vi "FEA_Model_Eigensolution.vi"(8 "error in (no error)":errorcluster, 11 "FEA_Model in":refnum<class "FEA_Model.lvclass">) -> (0 "error out":errorcluster, 3 "FEA_Model out":refnum<class "FEA_Model.lvclass">)   [LabVIEW 2021, in "FEA_Model.lvclass"]
uses:
  FEA_Model.lvclass
  FEA_Model.lvclass/FEA_Model.ctl
  <vilib>/Analysis/7linalg.llb/Eigenvalue and Vectors Output Option.ctl
  <vilib>/Analysis/baseanly.llb/Matrix Type of Inverse Matrix.ctl
  <vilib>/Analysis/7linalg.llb/Real Cholesky Factorization.vi
  <vilib>/Analysis/7linalg.llb/Real Generalized Eigenvalues and Vectors.vi
  <vilib>/Analysis/baseanly.llb/Full Cholesky Factorization.vi
  <vilib>/Analysis/baseanly.llb/Full Real Matrix Cholesky Factorization.vi
  <vilib>/Analysis/Matrix/Numeric/Conversions/Array To Matrix - RA2.vi
  <vilib>/Analysis/baseanly.llb/Real Inverse Matrix.vi
  <vilib>/Analysis/Matrix/Numeric/Multiply/Multiply - RM,RM.vi
  <vilib>/Analysis/Matrix/Numeric/Add/Add - RM,RM.vi
  <vilib>/Analysis/7linalg.llb/Real Eigenvalues and Vectors.vi
  <vilib>/Analysis/NI_AALPro.lvlib
  <vilib>/Analysis/Matrix/NI_Matrix.lvlib
  <vilib>/Analysis/NI_AALBase.lvlib
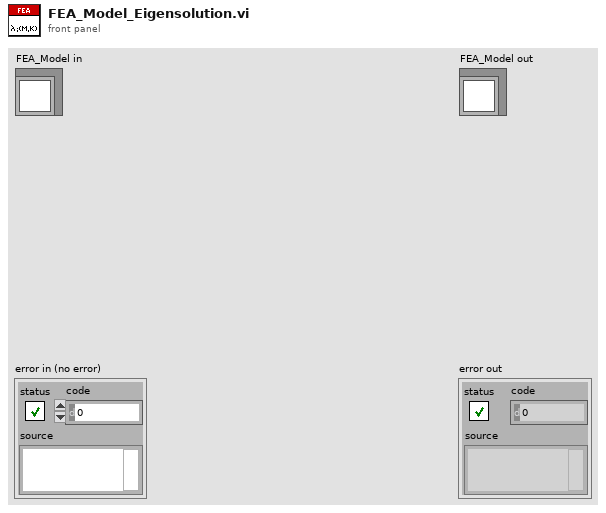
[diagram p1: front panel]
types:
  T1 = typedef "NI_AALBase.lvlib/Matrix Type of Inverse Matrix.ctl" = enum32{"General", "Positive Definite", "Lower Triangular", "Upper Triangular"}
  T2 = enum16{"LabVIEW Cholesky", "LabVIEW General", "LabVIEW Inverse", "LEMP"}
  T3 = typedef "NI_AALPro.lvlib/Eigenvalue and Vectors Output Option.ctl" = i32
  T4 = typedef "NI_Matrix.lvlib/RealMatrix.ctl" = dbl[][]
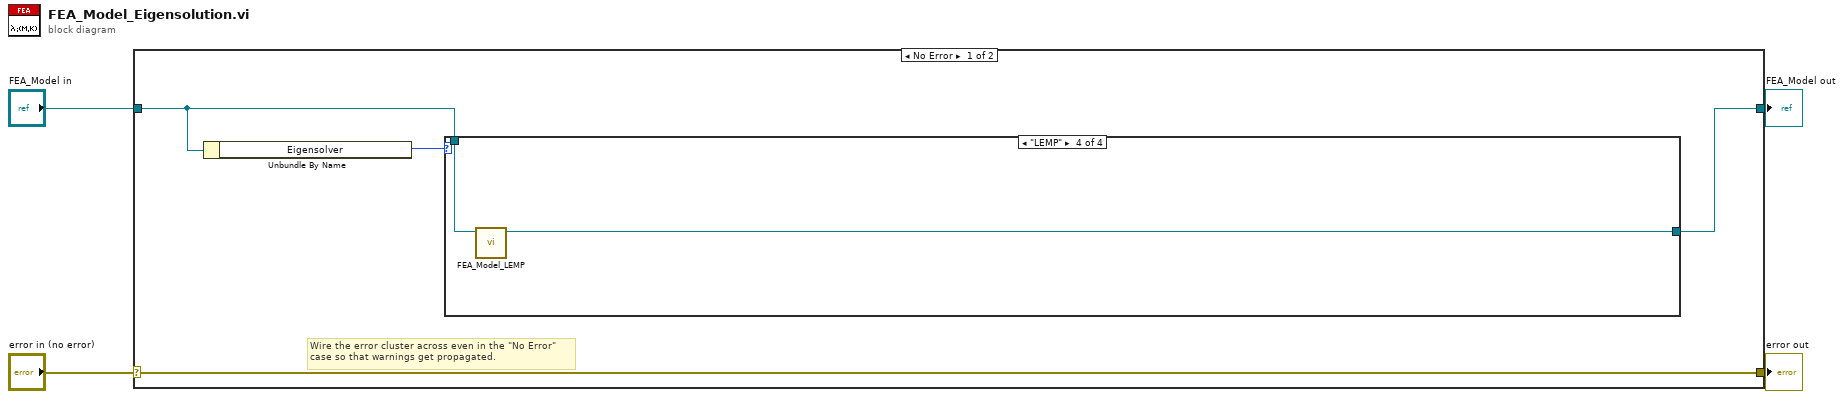
[diagram p0: block diagram]
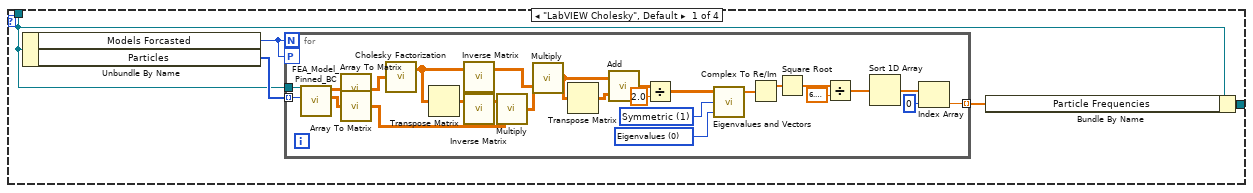
[diagram p2: hidden frame]
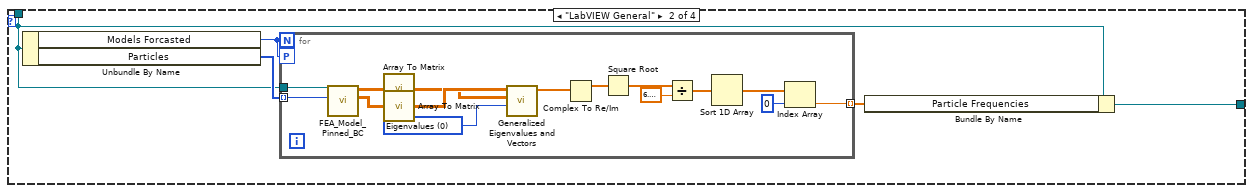
[diagram p3: hidden frame]
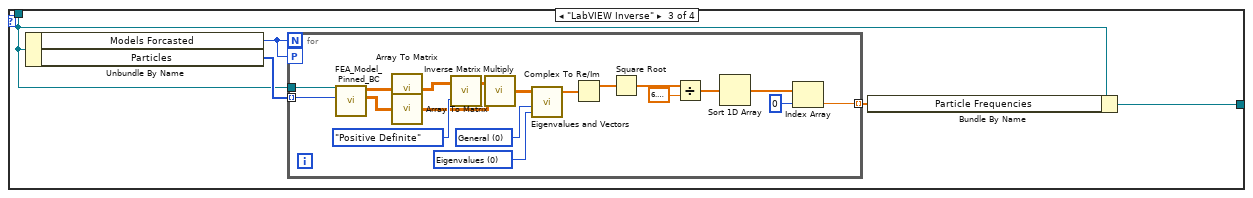
[diagram p4: hidden frame]
diagram:
  n1 = case shown="No Error" "error in (no error)" {
    selector: "error in (no error)" -> [w8 w87]
    tunnel: [w8 w87] -> w3
    tunnel: [w6 w86] -> w1
    tunnel: "FEA_Model in" -> [w5 w86]
    frame No Error {
      # "Wire the error cluster across even in the \"No Error\"\ncase so that warnings get propagated."
      n2 = Unbundle By Name(w5) -> ("Eigensolver"=w7:T2)
      n3 = case shown="\"LEMP\"" w7 {
        tunnel: [w10 w42 w61 w85] -> w6
        tunnel: w5 -> [w9 w40 w60 w84]
        frame "LabVIEW Cholesky", Default {
          n4 = Unbundle By Name(w9) -> ("Models Forcasted"=w13:i32, "Particles"=w12:i32[])
          n5 = for {
            N: w13 -> [_]
            workers-P: w13 -> [_]
            tunnel: w9 -> [w39]
            tunnel: w12 -> [w38] mode=indexing
            tunnel: [w29] -> w11 mode=indexing
            w18 = T3 0 items=["Eigenvalues", "Eigenvalues & Vectors"] ("output option")
            w19 = 1 items=["General", "Symmetric"] ("matrix type")
            n6 = call "FEA_Model_Pinned_BC.vi"("Pin Location"=w38, "FEA_Model in"=w39) -> ("K Matrix"=w36:dbl[][], "M Matrix"=w37:dbl[][])  [unwired: 8 in]
            n7 = call-poly <vilib>:"Array To Matrix.vi"("Real 2D Array"=w37) -> ("Real Matrix"=w16:T4)
            n8 = call-poly <vilib>:"Array To Matrix.vi"("Real 2D Array"=w36) -> ("Real Matrix"=w15:T4)
            n9 = call-poly <vilib>:"Cholesky Factorization.vi"("A"=w16) -> ("Cholesky"=w27:T4)  [unwired: 1 out]
            n10 = Transpose Matrix(1:w27) -> (0:w28:T4)
            n11 = call-poly <vilib>:"Inverse Matrix.vi"("Input Matrix"=w27) -> ("Inverse Matrix"=w25:T4)  [unwired: 1 in, 1 out]
            n12 = call-poly <vilib>:"Inverse Matrix.vi"("Input Matrix"=w28) -> ("Inverse Matrix"=w26:T4)  [unwired: 1 in, 1 out]
            n13 = call-poly <vilib>:"Multiply.vi"("Real Matrix B"=w15, "Real Matrix A"=w26) -> ("A * B"=w24:T4)
            n14 = call-poly <vilib>:"Multiply.vi"("Real Matrix B"=w25, "Real Matrix A"=w24) -> ("A * B"=w23:T4)
            n15 = Transpose Matrix(1:w23) -> (0:w22:T4)
            n16 = call-poly <vilib>:"Add.vi"("Real Matrix B"=w22, "Real Matrix A"=w23) -> ("A + B"=w20:T4)
            n17 = Divide(x=w20, y=2.0) -> (x/y=w17:T4)
            n18 = call-poly <vilib>:"Eigenvalues and Vectors.vi"("output option"=w18, "matrix type"=w19, "Input Matrix"=w17) -> ("Eigenvalues"=w14:cdb[])  [unwired: 2 out]
            n19 = Complex To Re/Im ("Complex To Cartesian.vi")(x + iy=w14) -> (x=w35:dbl[])  [unwired: 1 out]
            n20 = Square Root ("Square Root.vi")(x=w35) -> (sqrt(x)=w34:dbl[])
            n21 = Divide(x=w34, y=6.283185307179586) -> (x/y=w30:dbl[])
            n22 = Sort 1D Array(array=w30) -> (sorted array=w32:dbl[])
            n23 = Index Array(array=w32, index=0) -> (element=w29:dbl)
          }
          n24 = Bundle By Name(cluster=w9, "Particle Frequencies"=w11) -> (w10:refnum<class "FEA_Model.lvclass">)
        }
        frame "LabVIEW General" {
          n25 = Unbundle By Name(w40) -> ("Models Forcasted"=w44:i32, "Particles"=w43:i32[])
          n26 = for {
            N: w44 -> [_]
            workers-P: w44 -> [_]
            tunnel: w40 -> [w56]
            tunnel: w43 -> [w55] mode=indexing
            tunnel: [w45] -> w41 mode=indexing
            w59 = T3 0 items=["Eigenvalues", "Eigenvalues & Vectors"] ("output option")
            n27 = call "FEA_Model_Pinned_BC.vi"("Pin Location"=w55, "FEA_Model in"=w56) -> ("K Matrix"=w53:dbl[][], "M Matrix"=w54:dbl[][])  [unwired: 8 in]
            n28 = call-poly <vilib>:"Array To Matrix.vi"("Real 2D Array"=w54) -> ("Real Matrix"=w57:T4)
            n29 = call-poly <vilib>:"Array To Matrix.vi"("Real 2D Array"=w53) -> ("Real Matrix"=w58:T4)
            n30 = call-poly <vilib>:"Generalized Eigenvalues and Vectors.vi"("output option"=w59, "B"=w57, "A"=w58) -> ("Eigenvalues"=w46:cdb[])  [unwired: 3 in, 2 out]
            n31 = Complex To Re/Im ("Complex To Cartesian.vi")(x + iy=w46) -> (x=w52:dbl[])  [unwired: 1 out]
            n32 = Square Root ("Square Root.vi")(x=w52) -> (sqrt(x)=w51:dbl[])
            n33 = Divide(x=w51, y=6.283185307179586) -> (x/y=w47:dbl[])
            n34 = Sort 1D Array(array=w47) -> (sorted array=w49:dbl[])
            n35 = Index Array(array=w49, index=0) -> (element=w45:dbl)
          }
          n36 = Bundle By Name(cluster=w40, "Particle Frequencies"=w41) -> (w42:refnum<class "FEA_Model.lvclass">)
        }
        frame "LabVIEW Inverse" {
          n37 = Unbundle By Name(w60) -> ("Models Forcasted"=w64:i32, "Particles"=w63:i32[])
          n38 = for {
            N: w64 -> [_]
            workers-P: w64 -> [_]
            tunnel: w60 -> [w83]
            tunnel: w63 -> [w82] mode=indexing
            tunnel: [w73] -> w62 mode=indexing
            w69 = T3 0 items=["Eigenvalues", "Eigenvalues & Vectors"] ("output option")
            w71 = 0 items=["General", "Symmetric"] ("matrix type")
            n39 = call "FEA_Model_Pinned_BC.vi"("Pin Location"=w82, "FEA_Model in"=w83) -> ("K Matrix"=w80:dbl[][], "M Matrix"=w81:dbl[][])  [unwired: 8 in]
            n40 = call-poly <vilib>:"Array To Matrix.vi"("Real 2D Array"=w81) -> ("Real Matrix"=w66:T4)
            n41 = call-poly <vilib>:"Array To Matrix.vi"("Real 2D Array"=w80) -> ("Real Matrix"=w67:T4)
            n42 = call-poly <vilib>:"Inverse Matrix.vi"("matrix type"=Matrix_Type_of_Inverse_Matrix."Positive Definite", "Input Matrix"=w66) -> ("Inverse Matrix"=w72:T4)  [unwired: 1 out]
            n43 = call-poly <vilib>:"Multiply.vi"("Real Matrix B"=w67, "Real Matrix A"=w72) -> ("A * B"=w70:T4)
            n44 = call-poly <vilib>:"Eigenvalues and Vectors.vi"("output option"=w69, "matrix type"=w71, "Input Matrix"=w70) -> ("Eigenvalues"=w65:cdb[])  [unwired: 2 out]
            n45 = Complex To Re/Im ("Complex To Cartesian.vi")(x + iy=w65) -> (x=w79:dbl[])  [unwired: 1 out]
            n46 = Square Root ("Square Root.vi")(x=w79) -> (sqrt(x)=w78:dbl[])
            n47 = Divide(x=w78, y=6.283185307179586) -> (x/y=w74:dbl[])
            n48 = Sort 1D Array(array=w74) -> (sorted array=w76:dbl[])
            n49 = Index Array(array=w76, index=0) -> (element=w73:dbl)
          }
          n50 = Bundle By Name(cluster=w60, "Particle Frequencies"=w62) -> (w61:refnum<class "FEA_Model.lvclass">)
        }
        frame "LEMP" {
          n51 = call-dynamic "FEA_Model_LEMP.vi"("FEA_Model in"=w84) -> ("FEA_Model out"=w85:refnum<class "FEA_Model.lvclass">)  [unwired: 9 in, 1 out]
        }
      }
    }
    frame Error {
    }
  }
  "error out" <- w3
  "FEA_Model out" <- w1
